vi "PROXY_set_IP_and_port_after_connection_established.vi"(6 "station":T1, 8 "error_in":errorcluster, 10 "PLC_port":u16, 11 "PLC_IP":string) -> (0 "error_out":errorcluster)   [LabVIEW 2020]
uses:
  STATION/station.ctl
  FGV/DIAGNOSTICS_records_display/FGV_PROXY_DIAGNOSTICS_records_display.ctl
  _misc/PLC_connection_status.ctl
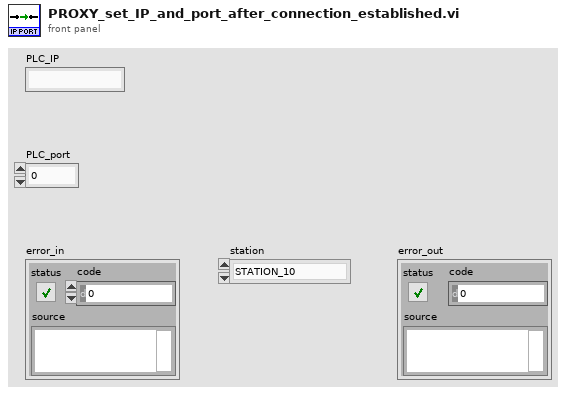
[diagram p1: front panel]
types:
  T1 = typedef "station.ctl" = enum16{"STATION_10", "STATION_20", "STATION_30", "STATION_40", "STATION_50", "STATION_60", "STATION_70", "STATION_80", "STATION_90", "STATION_100", "STATION_110", "STATION_120", "STATION_165", "MAIN"}
  T2 = typedef "PLC_connection_status.ctl" = enum16{"Connected", "Waiting", "Error", "-"}
  T3 = typedef "FGV_PROXY_DIAGNOSTICS_records_display.ctl" = enum16{"initialize", "set_PLC_IP", "set_PLC_Port", "set_PLC_connection_status", "set_SQL_connection_status", "get_all_info"}
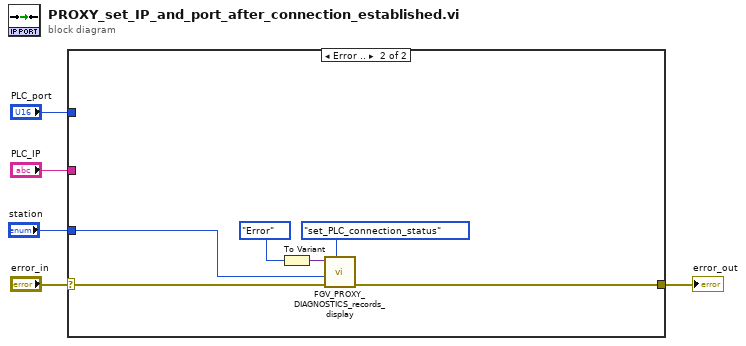
[diagram p0: block diagram]
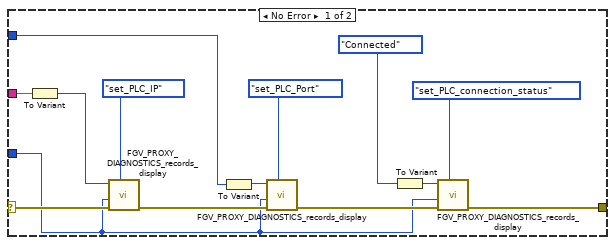
[diagram p2: hidden frame]
diagram:
  n1 = case shown="Error .." "error_in" {
    selector: "error_in" -> [w10 w22]
    tunnel: "PLC_port" -> [w16 _]
    tunnel: "PLC_IP" -> [w13 _]
    tunnel: [w7 w21] -> w2
    tunnel: "station" -> [w6 w20]
    frame No Error {
      n2 = To Variant(anything=w13) -> (Variant=w12:variant)
      n3 = call "FGV_PROXY_DIAGNOSTICS_records_display.vi"("options"=FGV_PROXY_DIAGNOSTICS_records_display."set_PLC_IP", "error_in"=w10, "station"=w6, "input"=w12) -> ("error_out"=w9:errorcluster)  [unwired: 6 in, 1 out]
      n4 = To Variant(anything=w16) -> (Variant=w15:variant)
      n5 = call "FGV_PROXY_DIAGNOSTICS_records_display.vi"("options"=FGV_PROXY_DIAGNOSTICS_records_display."set_PLC_Port", "error_in"=w9, "station"=w6, "input"=w15) -> ("error_out"=w8:errorcluster)  [unwired: 6 in, 1 out]
      n6 = To Variant(anything=PLC_connection_status."Connected" ("connection_status")) -> (Variant=w17:variant)
      n7 = call "FGV_PROXY_DIAGNOSTICS_records_display.vi"("options"=FGV_PROXY_DIAGNOSTICS_records_display."set_PLC_connection_status", "error_in"=w8, "station"=w6, "input"=w17) -> ("error_out"=w7:errorcluster)  [unwired: 6 in, 1 out]
    }
    frame Error {
      n8 = To Variant(anything=PLC_connection_status."Error" ("connection_status")) -> (Variant=w23:variant)
      n9 = call "FGV_PROXY_DIAGNOSTICS_records_display.vi"("options"=FGV_PROXY_DIAGNOSTICS_records_display."set_PLC_connection_status", "error_in"=w22, "station"=w20, "input"=w23) -> ("error_out"=w21:errorcluster)  [unwired: 6 in, 1 out]
    }
  }
  "error_out" <- w2
